vi "VOLT_CURRENT_COMMAND_MAKER.vi"(6 "Input value":dbl, 9 "Channel":u16, 10 "Measure (OUTPUT)":enum16{"Voltage", "Current"}(ring), 11 "Source":enum16{"Voltage", "Current"}(ring)) -> (3 "created command":string)   [LabVIEW 2020]
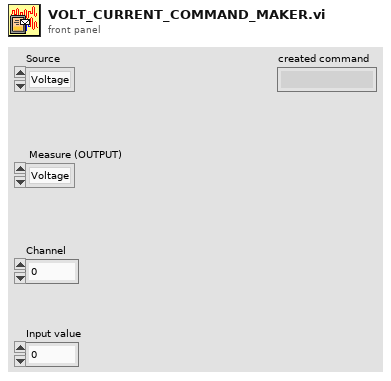
[diagram p1: front panel]
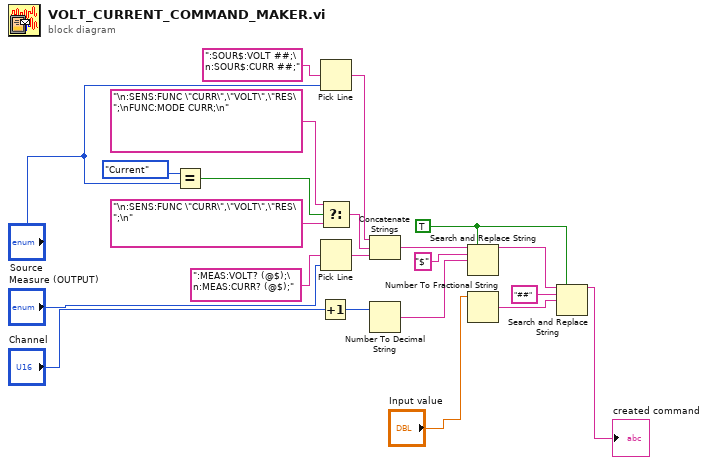
[diagram p0: block diagram]
diagram:
  w13 = TRUE ("replace all? (F)")
  n1 = Equal?(x=enum16{"Voltage", "Current"}."Current", y="Source") -> (x = y?=w17:bool)
  n2 = Increment(x="Channel") -> (x+1=w9:u16)
  n3 = Pick Line(multi-line string=":SOUR$:VOLT ##;\n:SOUR$:CURR ##;", line index="Source") -> (output string=w6:string)  [unwired: 1 in]
  n4 = Select(t="\n:SENS:FUNC \"CURR\",\"VOLT\",\"RES\";\nFUNC:MODE CURR;\n" ("string"), s=w17, f="\n:SENS:FUNC \"CURR\",\"VOLT\",\"RES\";\n") -> (s? t:f=w19:string)
  n5 = Pick Line(multi-line string=":MEAS:VOLT? (@$);\n:MEAS:CURR? (@$);", line index="Measure (OUTPUT)") -> (output string=w5:string)  [unwired: 1 in]
  n6 = Concatenate Strings(w6, w19, w5) -> (w7:string)
  n7 = Number To Decimal String(number=w9) -> (decimal integer string=w10:string)  [unwired: 1 in]
  n8 = Search and Replace String(replace all?=w13, input string=w7, search string="$", replace string=w10) -> (result string=w11:string)  [unwired: 4 in, 3 out]
  n9 = Number To Fractional String(number="Input value") -> (F-format string=w14:string)  [unwired: 3 in]
  n10 = Search and Replace String(replace all?=w13, input string=w11, search string="##", replace string=w14) -> (result string=→"created command":string)  [unwired: 4 in, 3 out]
